vi "DisconnectFromTypedefRecursive.vi"(8 "error in (no error)":errorcluster, 11 "VI ref (typedef)":refnum<vi>) -> (0 "error out":errorcluster, 3 "VI ref (typedef)":refnum<vi>)   [LabVIEW 2019, in "BlueUtilityScripts.lvlib"]
uses:
  BlueUtilityScripts.lvlib
  <vilib>/Utility/traverseref.llb/TRef TravTarget.ctl
  <vilib>/Utility/traverseref.llb/VI Scripting - Traverse.lvlib
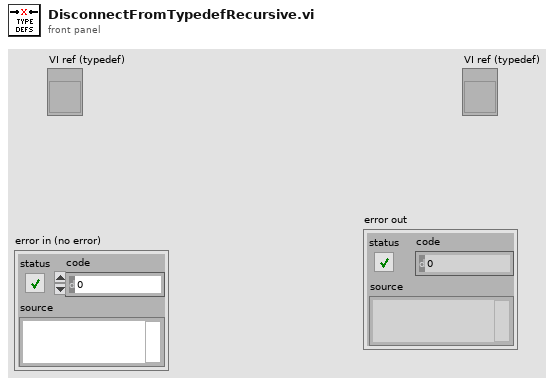
[diagram p1: front panel]
types:
  T1 = typedef "TRef TravTarget.ctl" = enum16{"FP", "BD", "Other"}
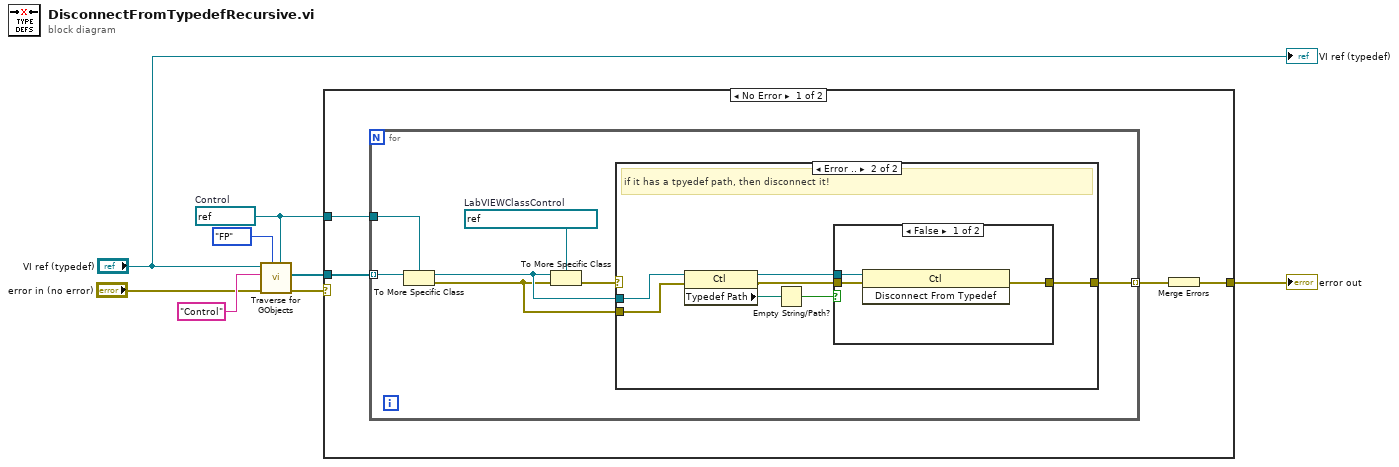
[diagram p0: block diagram]
diagram:
  w4 = refnum<vi> refnum  # Control
  n1 = call <vilib>:"Traverse for GObjects.vi"("Other Refnum"=w4, "Traverse Target"=TRef_TravTarget."FP", "error in (no error)"="error in (no error)", "Class Name"="Control", "VI Refnum"="VI ref (typedef)") -> ("error out"=w2:errorcluster, "References"=w5:refnum<vi>[])  [unwired: 3 in, 2 out]
  n2 = case shown="No Error" w2 {
    selector: w2 -> [_ w31]
    tunnel: w5 -> [w12 _]
    tunnel: w4 -> [w11 _]
    tunnel: [w9 w31] -> w3
    frame No Error {
      n3 = for {
        tunnel: [w17] -> w10 mode=indexing
        tunnel: w12 -> [w19] mode=indexing
        tunnel: w11 -> [w18]
        w16 = refnum<vi> refnum  # LabVIEWClassControl
        n4 = To More Specific Class(target class=w18, reference=w19) -> (specific class reference=w14:refnum<vi>, error out=w13:errorcluster)  [unwired: 1 in]
        n5 = To More Specific Class(target class=w16, reference=w14, error in=w13) -> (error out=w15:errorcluster)  [unwired: 1 out]
        n6 = case shown="Error .." w15 {
          tunnel: [_ w26] -> w17
          tunnel: w14 -> [_ w21]
          tunnel: w13 -> [_ w20]
          frame No Error {
            # "Don't disconnect LabVIEW Class Controls"
          }
          frame Error {
            # "if it has a tpyedef path, then disconnect it!"
            n7 = property class="Ctl"(reference=w21, error in=w20) -> (reference out=w24:refnum<vi>, error out=w23:errorcluster, "Typedef Path"=w25:path)
            n8 = Empty String/Path?(string/path=w25) -> (empty?=w22:bool)
            n9 = case shown="False" w22 {
              tunnel: [w29 w30] -> w26
              tunnel: w24 -> [w28 _]
              tunnel: w23 -> [w27 w30]
              frame False {
                n10 = invoke class="Ctl" method="Disconnect From Typedef"(reference=w28, error in=w27) -> (error out=w29:errorcluster)  [unwired: 1 in, 2 out]
              }
              frame True {
              }
            }
          }
        }
      }
      n11 = Merge Errors(w10) -> (w9:errorcluster)
    }
    frame Error {
    }
  }
  "error out" <- w3
  "VI ref (typedef)" <- "VI ref (typedef)"
